vi "RichToFlatnixnet_grpc_U32Array.vi"(5 "OutputClusterType":T1, 11 "InputCluster":T2) -> (3 "OutputCluster":T1)   [LabVIEW 2024, in "grpc-xnet_client.lvlib"]
uses:
  grpc-xnet_client.lvlib
  nixnet_grpc_U32Array_Flat.ctl
  nixnet_grpc_U32Array.ctl
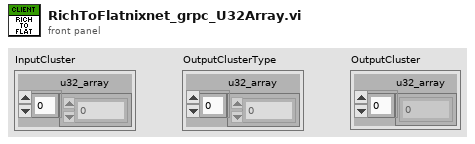
[diagram p1: front panel]
types:
  T1 = typedef "grpc-xnet_client.lvlib/nixnet_grpc_U32Array_Flat.ctl" = cluster{"u32_array":u32[]}
  T2 = typedef "grpc-xnet_client.lvlib/nixnet_grpc_U32Array.ctl" = cluster{"u32_array":u32[]}
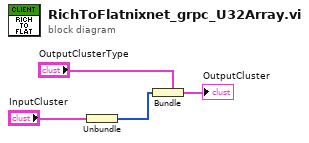
[diagram p0: block diagram]
diagram:
  n1 = Unbundle "Unbundle"("InputCluster") -> ("u32_array"=w1:u32[])
  n2 = Bundle "Bundle"(cluster="OutputClusterType", "u32_array"=w1) -> (→"OutputCluster":T1)
